vi "OX v1.2.vi"(2 "INDICATOR INPUT":dbl[](array[numeric]), 3 "DATA INPUT":dbl[](array[numeric])) -> (0 "OUTPUT":dbl[][](array[numeric]))   [LabVIEW 2019]
uses:
  <vilib>/ptbypt/NI_PtbyPt.lvlib
panel:
  in  "FU BUTTON FEEDBACK":dbl[](array[numeric])
  out "PH LED 6":bool=TRUE
  in  "PH CHECK 6":bool
  out "PH IND 6":bool=TRUE
  out "PH LED 5":bool=TRUE
  out "PH LED 4":bool=TRUE
  out "PH LED 3":bool=TRUE
  out "PH LED 2":bool=TRUE
  out "PH LED 1":bool=TRUE
  in  "PH CHECK 1":bool
  in  "PH CHECK 2":bool
  in  "PH CHECK 3":bool
  in  "PH CHECK 4":bool
  in  "PH CHECK 5":bool
  out "PH IND 5":bool=TRUE
  out "PH IND 4":bool=TRUE
  out "PH IND 3":bool=TRUE
  out "PH IND 2":bool=TRUE
  out "PH IND 1":bool=TRUE
  out "STARTUP GNG":bool=TRUE
  out "STARTUP GNG NUM":dbl
  out "STARTUP GNG LED":bool=TRUE
  out "CHILL GNG":bool=TRUE
  out "CHILL GNG NUM":dbl
  out "CHILL GNG LED":bool=TRUE
  out "OX ISO GNG":bool=TRUE
  out "OX ISO GNG NUM":dbl
  out "OX ISO GNG LED":bool=TRUE
  out "RECORD GNG":bool=TRUE
  out "RECORD GNG NUM":dbl
  out "RECORD GNG LED":bool=TRUE
  out "OX VENT GNG":bool=TRUE
  out "OX VENT GNG NUM":dbl
  out "OX VENT GNG LED":bool=TRUE
  out "OX CHILL LINE TEMP":dbl(slide) scale=-200.0..75.0
  out "OX CHILL RELIEF TEMP":dbl(slide) scale=-200.0..75.0
  out "OX TANK TEMP 4":dbl
  out "OX TANK TEMP 3":dbl
  out "OX TANK TEMP 2":dbl
  out "OX TANK TEMP 1":dbl
  out "OX MAIN VALVE TEMP":dbl(slide) scale=-200.0..75.0
  out "OX VENTURI TEMP":dbl(slide) scale=-200.0..75.0
  out "TANK TEMP CB 1":u32(colorbox)
  out "TANK TEMP CB 2":u32(colorbox)
  out "TANK TEMP CB 3":u32(colorbox)
  out "TANK TEMP CB 4":u32(colorbox)
  out "OX MAIN LINE TEMP":dbl(slide) scale=-200.0..75.0
  out "SUB PANELS GNG":bool=TRUE
  out "SUB PANEL OX GNG NUM":dbl
  out "SUB PANEL OX GNG LED":bool=TRUE
  out "VALVE STATES GNG":bool=TRUE
  out "VALVE ST OX GNG NUM":dbl
  out "VALVE ST OX GNG LED":bool=TRUE
  out "PRESS VALVES GNG":bool=TRUE
  out "PRESS VALVE OX GNG NUM":dbl
  out "PRESS VALVE OX GNG LED":bool=TRUE
  out "ARM GNG":bool=TRUE
  out "IGN TRIPPED GNG":bool=TRUE
  out "ARMED GNG NUM":dbl
  out "ARMED GNG LED":bool=TRUE
  out "IGN TRIPPED GNG NUM":dbl
  out "IGN TRIPPED GNG LED":bool=TRUE
  in  "Ox GNG BUTTON":bool
  out "OX GNG MAIN LED":bool=TRUE
  in  "ABORT BUTTON":bool
  out "ARMED PANEL LED":bool
  out "IGN INSERTED PANEL LED":bool
  out "NANNY PAN LED":bool
  out "SYS STATUS MAIN STRING":string
  out "REG PRESS GNG":bool=TRUE
  out "RELIEF GNG":bool=TRUE
  out "REG PRESS OX GNG NUM":dbl
  out "REG PRESS OX GNG LED":bool=TRUE
  out "RELIEF OX GNG NUM":dbl
  out "RELIEF OX GNG LED":bool=TRUE
  out "TANK PRESS GNG":bool=TRUE
  out "TANK PRESS OX GNG NUM":dbl
  out "TANK PRESS OX GNG LED":bool=TRUE
  out "FILL VALVES GNG":bool=TRUE
  out "FILL VALVE OX GNG NUM":dbl
  out "FILL VALVE OX GNG LED":bool=TRUE
  out "TANK LEVEL GNG":bool=TRUE
  out "TANK LEVEL OX GNG NUM":dbl
  out "TANK LEVEL OX GNG LED":bool=TRUE
  out "OX TANK RELIEF TEMP":dbl(slide) scale=-200.0..75.0
  out "MAIN PRESS OX METER":dbl(knob) scale=0.0..1600.0
  out "MAIN LINE PRESS OX METER":dbl(knob) scale=0.0..1600.0
  out "TANK PRESS OX METER":dbl(knob) scale=0.0..1600.0
  out "REG PRESS OX METER":dbl(knob) scale=0.0..1600.0
  out "Ox SYSTEM PRESSURE":dbl[](graph) caption="Waveform Chart - dark"
  out "FUEL TANK LEVEL (%)":dbl(slide) scale=0.0..100.0
  in  "ABV-OX-250  (Ox FILL)":bool
  out "OX FILL LED":bool=TRUE
  in  "ABV-OX-240 (Ox CHILL)":bool
  out "ABV-OX-240 LED":bool=TRUE
  in  "ABV-OX-230 (Ox MAIN)":bool
  out "ABV-OX-230 LED":bool=TRUE
  in  "ABV-OX-220 (Ox ISO)":bool
  out "ABV-OX-230 LED":bool=TRUE
  in  "ABV-OX-210 (Ox VENT)":bool
  out "ABV-OX-210 LED":bool=TRUE
  in  "ABV-OX-110 (Ox PRESS)":bool
  out "ABV-PR-110 LED":bool=TRUE
  # "Ox CONTROL"
  # "NANNY"
  # "IGNITOR \nINSERTED"
  # "ARMED"
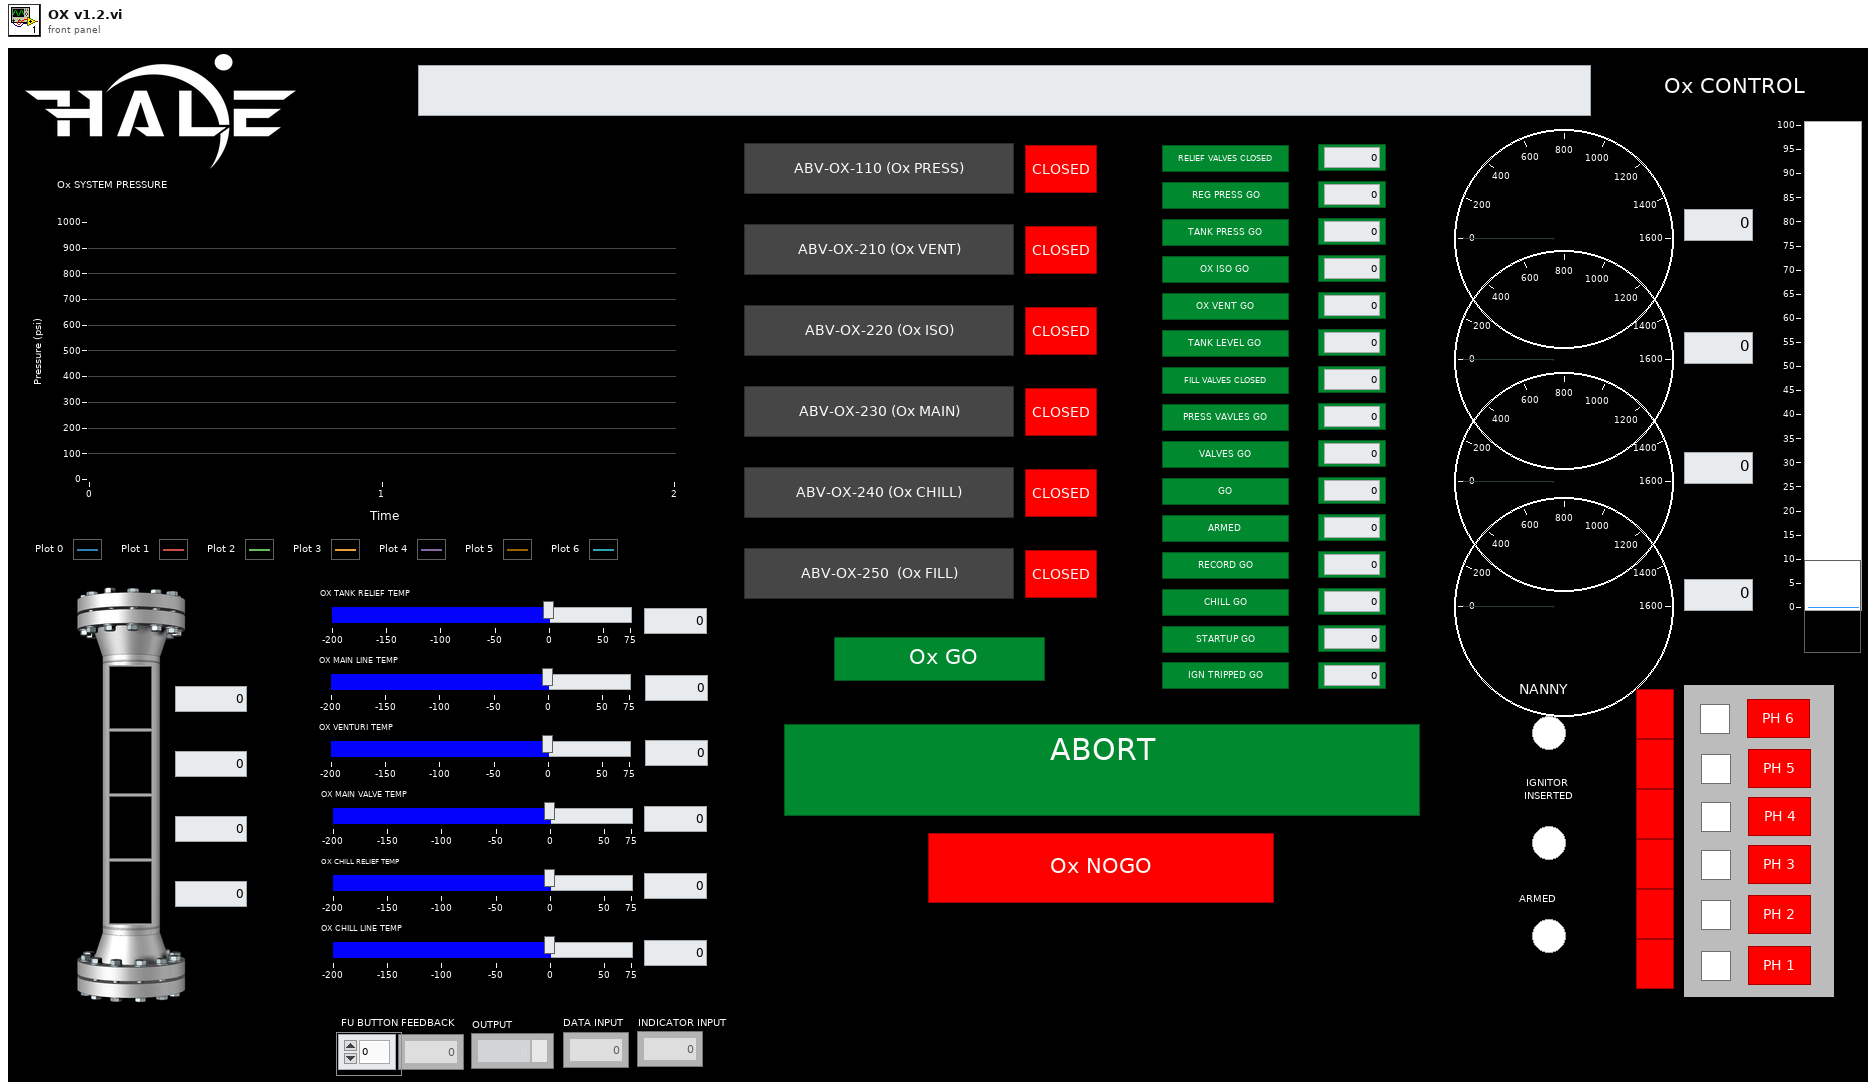
[diagram p1: front panel]
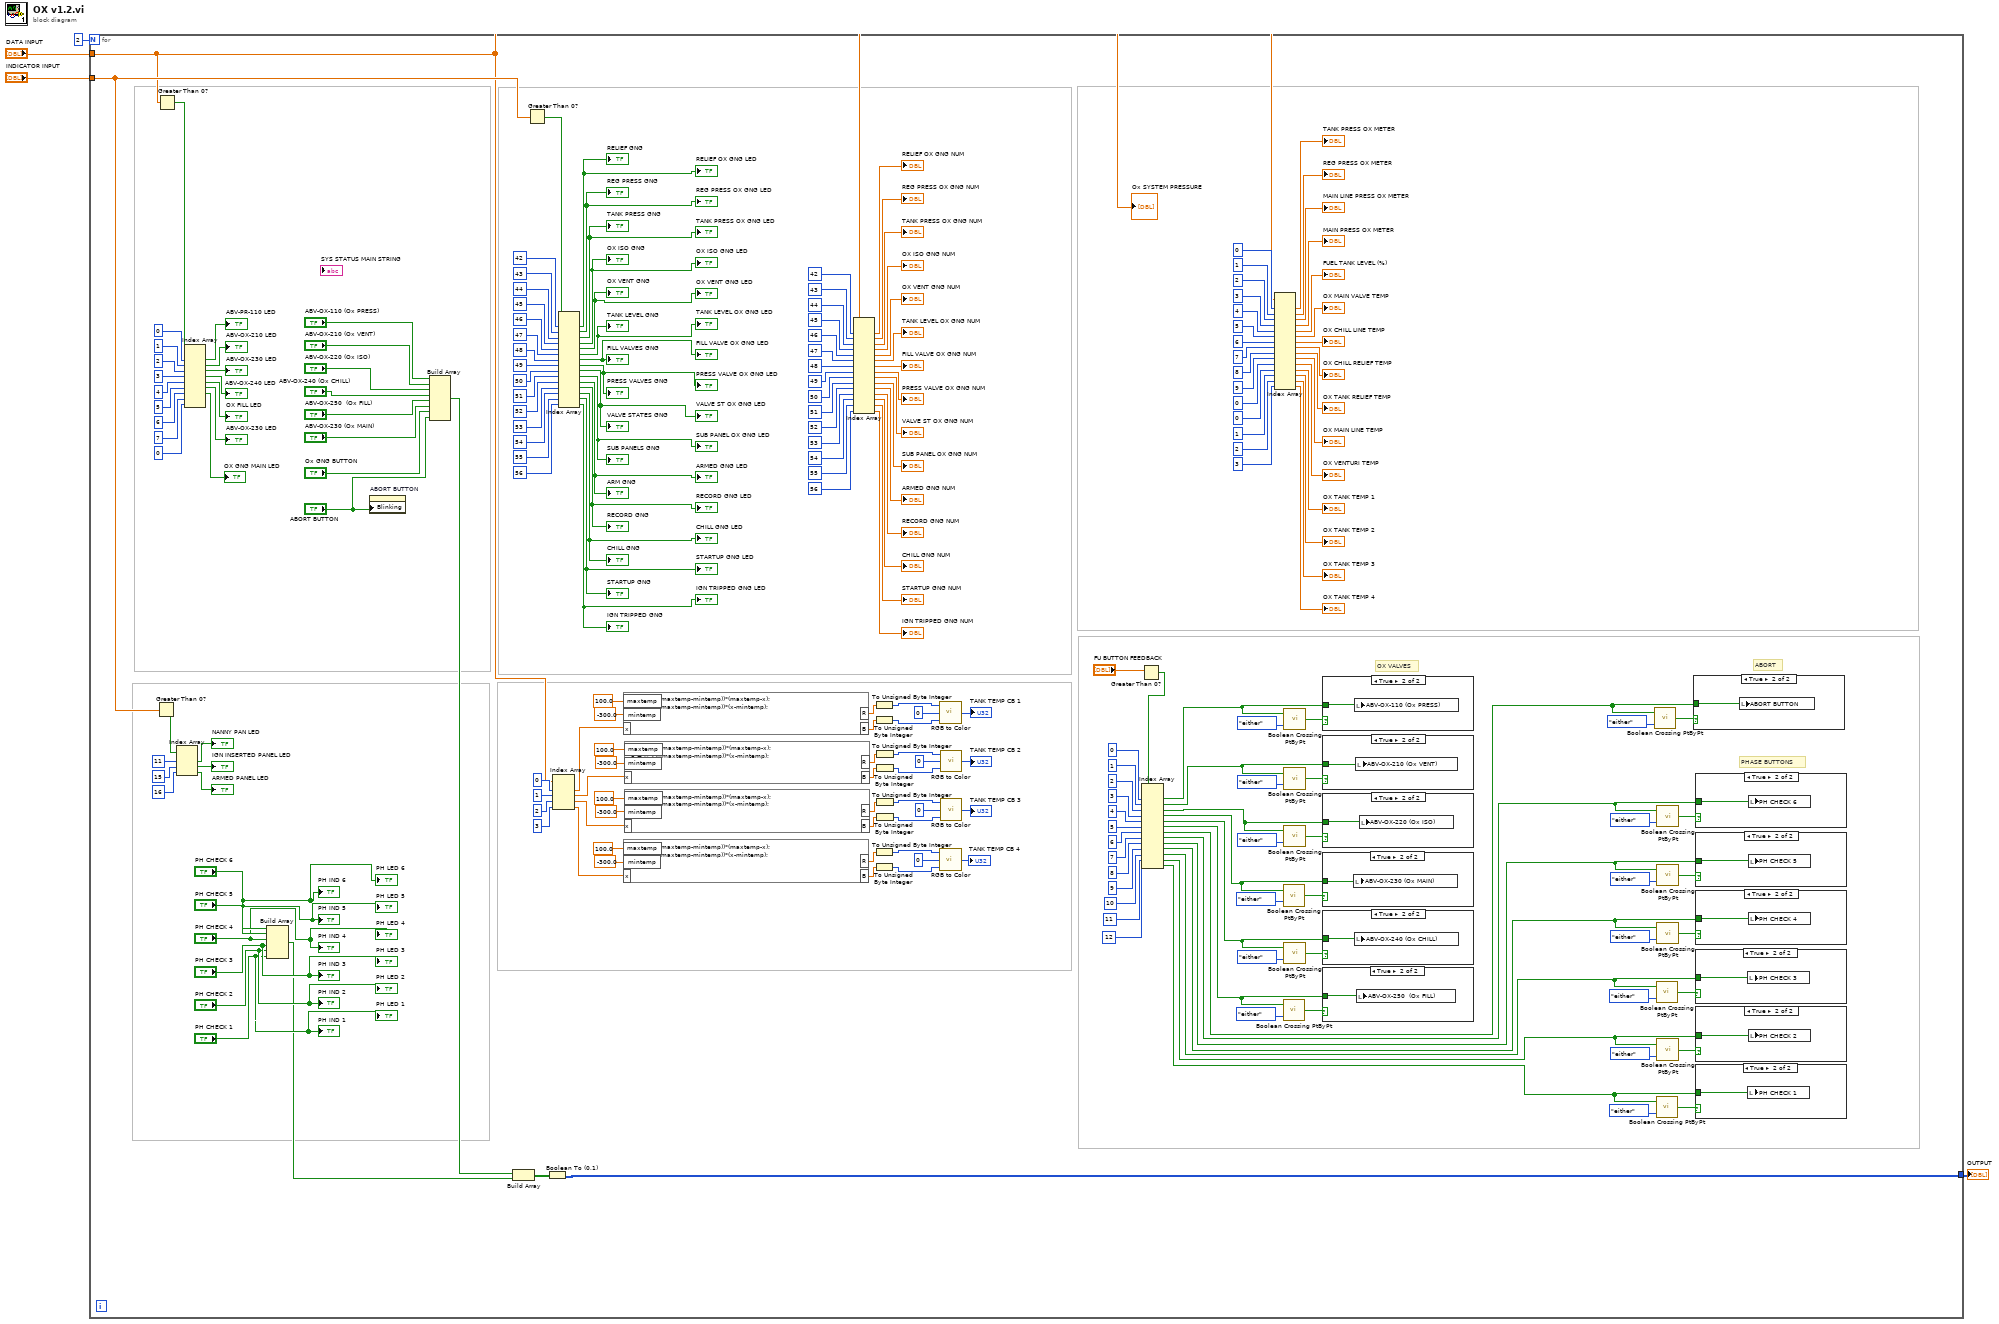
[diagram p0: block diagram]
diagram:
  n1 = for {
    N: 2 -> [_]
    tunnel: "INDICATOR INPUT" -> [w75]
    tunnel: "DATA INPUT" -> [w5]
    tunnel: [w64] -> w1
    # "ABORT"
    # "PHASE BUTTONS"
    # "OX VALVES"
    n2 = Greater Than 0?(x=w75) -> (x > 0?=w74:bool[])
    n3 = Greater Than 0?(x=w5) -> (x > 0?=w166:bool[])
    n4 = Index Array(array=w74, index #1=11 ("index"), index #2=15 ("index"), index #3=16 ("index")) -> (element #1=→"NANNY PAN LED":bool, element #2=→"IGN INSERTED PANEL LED":bool, element #3=→"ARMED PANEL LED":bool)
    n5 = Index Array(array=w166, index #1=0 ("index"), index #2=1 ("index"), index #3=2 ("index"), index #4=3 ("index"), index #5=4 ("index"), index #6=5 ("index"), index #7=6 ("index"), index #8=7 ("index"), index #9=0 ("index")) -> (element #1=→"ABV-PR-110 LED":bool, element #2=→"ABV-OX-210 LED":bool, element #3=→"ABV-OX-230 LED":bool, element #4=→"ABV-OX-240 LED":bool, element #5=→"OX FILL LED":bool, element #6=→"ABV-OX-230 LED":bool, element #7=→"OX GNG MAIN LED":bool)  [unwired: 2 out]
    n6 = Build Array("PH CHECK 6", "PH CHECK 5", "PH CHECK 4", "PH CHECK 3", "PH CHECK 2", "PH CHECK 1") -> (w66:bool[])
    n7 = property on="ABORT BUTTON" class="Bool (strict)"("Blinking"="ABORT BUTTON") -> ()  [unwired: 2 in, 2 out]
    n8 = Build Array("ABV-OX-110 (Ox PRESS)", "ABV-OX-210 (Ox VENT)", "ABV-OX-220 (Ox ISO)", "ABV-OX-240 (Ox CHILL)", "ABV-OX-250  (Ox FILL)", "ABV-OX-230 (Ox MAIN)", "Ox GNG BUTTON", "ABORT BUTTON") -> (w65:bool[])
    n9 = Build Array(w65, w66) -> (w67:bool[][])
    n10 = Greater Than 0?(x=w75) -> (x > 0?=w106:bool[])
    n11 = Boolean To (0,1)(Boolean=w67) -> (0, 1=w64:i16[][])
    n12 = Index Array(array=w5, index #1=0 ("index"), index #2=1 ("index"), index #3=2 ("index"), index #4=3 ("index")) -> (element #1=w114:dbl, element #2=w113:dbl, element #3=w112:dbl, element #4=w111:dbl)
    n13 = Index Array(array=w106, index #1=42 ("index"), index #2=43 ("index"), index #3=44 ("index"), index #4=45 ("index"), index #5=46 ("index"), index #6=47 ("index"), index #7=48 ("index"), index #8=49 ("index"), index #9=50 ("index"), index #10=51 ("index"), index #11=52 ("index"), index #12=53 ("index"), index #13=54 ("index"), index #14=55 ("index"), index #15=56 ("index")) -> (element #1=→"RELIEF OX GNG LED" →"RELIEF GNG":bool, element #2=→"REG PRESS OX GNG LED" →"REG PRESS GNG":bool, element #3=→"TANK PRESS OX GNG LED" →"TANK PRESS GNG":bool, element #4=→"OX ISO GNG LED" →"OX ISO GNG":bool, element #5=→"OX VENT GNG LED" →"OX VENT GNG":bool, element #6=→"TANK LEVEL OX GNG LED" →"TANK LEVEL GNG":bool, element #7=→"FILL VALVE OX GNG LED" →"FILL VALVES GNG":bool, element #8=→"PRESS VALVE OX GNG LED" →"PRESS VALVES GNG":bool, element #9=→"VALVE ST OX GNG LED" →"VALVE STATES GNG":bool, element #10=→"SUB PANEL OX GNG LED" →"SUB PANELS GNG":bool, element #11=→"ARMED GNG LED" →"ARM GNG":bool, element #12=→"RECORD GNG LED" →"RECORD GNG":bool, element #13=→"CHILL GNG LED" →"CHILL GNG":bool, element #14=→"STARTUP GNG LED" →"STARTUP GNG":bool, element #15=→"IGN TRIPPED GNG LED" →"IGN TRIPPED GNG":bool)
    n14 = formula code="B = (255/(maxtemp-mintemp))*(maxtemp-x);\nR = (255/(maxtemp-mintemp))*(x-mintemp);"("maxtemp"=100.0 ("input variable"), "mintemp"=-300.0 ("input variable"), "x"=w114) -> ("B"=w160:dbl, "R"=w162:dbl)
    n15 = formula code="B = (255/(maxtemp-mintemp))*(maxtemp-x);\nR = (255/(maxtemp-mintemp))*(x-mintemp);"("maxtemp"=100.0 ("input variable"), "mintemp"=-300.0 ("input variable"), "x"=w111) -> ("B"=w124:dbl, "R"=w126:dbl)
    n16 = formula code="B = (255/(maxtemp-mintemp))*(maxtemp-x);\nR = (255/(maxtemp-mintemp))*(x-mintemp);"("maxtemp"=100.0 ("input variable"), "mintemp"=-300.0 ("input variable"), "x"=w113) -> ("B"=w138:dbl, "R"=w140:dbl)
    n17 = formula code="B = (255/(maxtemp-mintemp))*(maxtemp-x);\nR = (255/(maxtemp-mintemp))*(x-mintemp);"("maxtemp"=100.0 ("input variable"), "mintemp"=-300.0 ("input variable"), "x"=w112) -> ("B"=w131:dbl, "R"=w133:dbl)
    n18 = Index Array(array=w5, index #1=42 ("index"), index #2=43 ("index"), index #3=44 ("index"), index #4=45 ("index"), index #5=46 ("index"), index #6=47 ("index"), index #7=48 ("index"), index #8=49 ("index"), index #9=50 ("index"), index #10=51 ("index"), index #11=52 ("index"), index #12=53 ("index"), index #13=54 ("index"), index #14=55 ("index"), index #15=56 ("index")) -> (element #1=→"RELIEF OX GNG NUM":dbl, element #2=→"REG PRESS OX GNG NUM":dbl, element #3=→"TANK PRESS OX GNG NUM":dbl, element #4=→"OX ISO GNG NUM":dbl, element #5=→"OX VENT GNG NUM":dbl, element #6=→"TANK LEVEL OX GNG NUM":dbl, element #7=→"FILL VALVE OX GNG NUM":dbl, element #8=→"PRESS VALVE OX GNG NUM":dbl, element #9=→"VALVE ST OX GNG NUM":dbl, element #10=→"SUB PANEL OX GNG NUM":dbl, element #11=→"ARMED GNG NUM":dbl, element #12=→"RECORD GNG NUM":dbl, element #13=→"CHILL GNG NUM":dbl, element #14=→"STARTUP GNG NUM":dbl, element #15=→"IGN TRIPPED GNG NUM":dbl)
    n19 = To Unsigned Byte Integer(number=w162) -> (unsigned 8bit integer=w161:u8)
    n20 = To Unsigned Byte Integer(number=w160) -> (unsigned 8bit integer=w159:u8)
    n21 = To Unsigned Byte Integer(number=w126) -> (unsigned 8bit integer=w125:u8)
    n22 = To Unsigned Byte Integer(number=w124) -> (unsigned 8bit integer=w123:u8)
    n23 = To Unsigned Byte Integer(number=w140) -> (unsigned 8bit integer=w139:u8)
    n24 = To Unsigned Byte Integer(number=w138) -> (unsigned 8bit integer=w137:u8)
    n25 = To Unsigned Byte Integer(number=w133) -> (unsigned 8bit integer=w132:u8)
    n26 = To Unsigned Byte Integer(number=w131) -> (unsigned 8bit integer=w130:u8)
    n27 = call <vilib>:"RGB to Color.vi"("B"=w159, "G"=u8 0, "R"=w161) -> ("Color"=→"TANK TEMP CB 1":u32)
    n28 = call <vilib>:"RGB to Color.vi"("B"=w123, "G"=u8 0, "R"=w125) -> ("Color"=→"TANK TEMP CB 4":u32)
    n29 = call <vilib>:"RGB to Color.vi"("B"=w137, "G"=u8 0, "R"=w139) -> ("Color"=→"TANK TEMP CB 2":u32)
    n30 = call <vilib>:"RGB to Color.vi"("B"=w130, "G"=u8 0, "R"=w132) -> ("Color"=→"TANK TEMP CB 3":u32)
    n31 = Greater Than 0?(x="FU BUTTON FEEDBACK") -> (x > 0?=w10:bool[])
    n32 = Index Array(array=w10, index #1=0 ("index"), index #2=1 ("index"), index #3=2 ("index"), index #4=3 ("index"), index #5=4 ("index"), index #6=5 ("index"), index #7=6 ("index"), index #8=7 ("index"), index #9=8 ("index"), index #10=9 ("index"), index #11=10 ("index"), index #12=11 ("index"), index #13=12 ("index")) -> (element #1=w25:bool, element #2=w24:bool, element #3=w23:bool, element #4=w22:bool, element #5=w21:bool, element #6=w20:bool, element #7=w19:bool, element #8=w18:bool, element #9=w17:bool, element #10=w16:bool, element #11=w15:bool, element #12=w14:bool, element #13=w13:bool)
    n33 = Index Array(array=w5, index #1=0 ("index"), index #2=1 ("index"), index #3=2 ("index"), index #4=3 ("index"), index #5=4 ("index"), index #6=5 ("index"), index #7=6 ("index"), index #8=7 ("index"), index #9=8 ("index"), index #10=9 ("index"), index #11=0 ("index"), index #12=0 ("index"), index #13=1 ("index"), index #14=2 ("index"), index #15=3 ("index")) -> (element #1=→"TANK PRESS OX METER":dbl, element #2=→"REG PRESS OX METER":dbl, element #3=→"MAIN LINE PRESS OX METER":dbl, element #4=→"MAIN PRESS OX METER":dbl, element #5=→"FUEL TANK LEVEL (%)":dbl, element #6=→"OX MAIN VALVE TEMP":dbl, element #7=→"OX CHILL LINE TEMP":dbl, element #8=→"OX CHILL RELIEF TEMP":dbl, element #9=→"OX TANK RELIEF TEMP":dbl, element #10=→"OX MAIN LINE TEMP":dbl, element #11=→"OX VENTURI TEMP":dbl, element #12=→"OX TANK TEMP 1":dbl, element #13=→"OX TANK TEMP 2":dbl, element #14=→"OX TANK TEMP 3":dbl, element #15=→"OX TANK TEMP 4":dbl)
    n34 = call <vilib>:"Boolean Crossing PtByPt.vi"("direction"=enum16{"either", "false-true", "true-false"}."either", "input"=w22) -> ("crossing"=w57:bool)  [unwired: 1 in]
    n35 = call <vilib>:"Boolean Crossing PtByPt.vi"("direction"=enum16{"either", "false-true", "true-false"}."either", "input"=w20) -> ("crossing"=w53:bool)  [unwired: 1 in]
    n36 = call <vilib>:"Boolean Crossing PtByPt.vi"("direction"=enum16{"either", "false-true", "true-false"}."either", "input"=w25) -> ("crossing"=w63:bool)  [unwired: 1 in]
    n37 = call <vilib>:"Boolean Crossing PtByPt.vi"("direction"=enum16{"either", "false-true", "true-false"}."either", "input"=w24) -> ("crossing"=w61:bool)  [unwired: 1 in]
    n38 = call <vilib>:"Boolean Crossing PtByPt.vi"("direction"=enum16{"either", "false-true", "true-false"}."either", "input"=w23) -> ("crossing"=w59:bool)  [unwired: 1 in]
    n39 = call <vilib>:"Boolean Crossing PtByPt.vi"("direction"=enum16{"either", "false-true", "true-false"}."either", "input"=w21) -> ("crossing"=w55:bool)  [unwired: 1 in]
    n40 = case shown="True" w57 {
      tunnel: w22 -> [_ w243]
      frame False {
      }
      frame True {
        n41 = local write "ABV-OX-230 (Ox MAIN)"(w243) -> ()
      }
    }
    n42 = case shown="True" w53 {
      tunnel: w20 -> [_ w241]
      frame False {
      }
      frame True {
        n43 = local write "ABV-OX-250  (Ox FILL)"(w241) -> ()
      }
    }
    n44 = case shown="True" w63 {
      tunnel: w25 -> [_ w246]
      frame False {
      }
      frame True {
        n45 = local write "ABV-OX-110 (Ox PRESS)"(w246) -> ()
      }
    }
    n46 = case shown="True" w61 {
      tunnel: w24 -> [_ w245]
      frame False {
      }
      frame True {
        n47 = local write "ABV-OX-210 (Ox VENT)"(w245) -> ()
      }
    }
    n48 = case shown="True" w59 {
      tunnel: w23 -> [_ w244]
      frame False {
      }
      frame True {
        n49 = local write "ABV-OX-220 (Ox ISO)"(w244) -> ()
      }
    }
    n50 = case shown="True" w55 {
      tunnel: w21 -> [_ w242]
      frame False {
      }
      frame True {
        n51 = local write "ABV-OX-240 (Ox CHILL)"(w242) -> ()
      }
    }
    n52 = call <vilib>:"Boolean Crossing PtByPt.vi"("direction"=enum16{"either", "false-true", "true-false"}."either", "input"=w19) -> ("crossing"=w39:bool)  [unwired: 1 in]
    n53 = call <vilib>:"Boolean Crossing PtByPt.vi"("direction"=enum16{"either", "false-true", "true-false"}."either", "input"=w15) -> ("crossing"=w45:bool)  [unwired: 1 in]
    n54 = call <vilib>:"Boolean Crossing PtByPt.vi"("direction"=enum16{"either", "false-true", "true-false"}."either", "input"=w13) -> ("crossing"=w41:bool)  [unwired: 1 in]
    n55 = call <vilib>:"Boolean Crossing PtByPt.vi"("direction"=enum16{"either", "false-true", "true-false"}."either", "input"=w18) -> ("crossing"=w51:bool)  [unwired: 1 in]
    n56 = call <vilib>:"Boolean Crossing PtByPt.vi"("direction"=enum16{"either", "false-true", "true-false"}."either", "input"=w17) -> ("crossing"=w49:bool)  [unwired: 1 in]
    n57 = call <vilib>:"Boolean Crossing PtByPt.vi"("direction"=enum16{"either", "false-true", "true-false"}."either", "input"=w16) -> ("crossing"=w47:bool)  [unwired: 1 in]
    n58 = call <vilib>:"Boolean Crossing PtByPt.vi"("direction"=enum16{"either", "false-true", "true-false"}."either", "input"=w14) -> ("crossing"=w43:bool)  [unwired: 1 in]
    n59 = case shown="True" w39 {
      tunnel: w19 -> [_ w234]
      frame False {
      }
      frame True {
        n60 = local write "ABORT BUTTON"(w234) -> ()
      }
    }
    n61 = case shown="True" w45 {
      tunnel: w15 -> [_ w237]
      frame False {
      }
      frame True {
        n62 = local write "PH CHECK 3"(w237) -> ()
      }
    }
    n63 = case shown="True" w41 {
      tunnel: w13 -> [_ w235]
      frame False {
      }
      frame True {
        n64 = local write "PH CHECK 1"(w235) -> ()
      }
    }
    n65 = case shown="True" w51 {
      tunnel: w18 -> [_ w240]
      frame False {
      }
      frame True {
        n66 = local write "PH CHECK 6"(w240) -> ()
      }
    }
    n67 = case shown="True" w49 {
      tunnel: w17 -> [_ w239]
      frame False {
      }
      frame True {
        n68 = local write "PH CHECK 5"(w239) -> ()
      }
    }
    n69 = case shown="True" w47 {
      tunnel: w16 -> [_ w238]
      frame False {
      }
      frame True {
        n70 = local write "PH CHECK 4"(w238) -> ()
      }
    }
    n71 = case shown="True" w43 {
      tunnel: w14 -> [_ w236]
      frame False {
      }
      frame True {
        n72 = local write "PH CHECK 2"(w236) -> ()
      }
    }
    "Ox SYSTEM PRESSURE" <- w5
    "PH IND 1" <- "PH CHECK 1"
    "PH IND 2" <- "PH CHECK 2"
    "PH IND 3" <- "PH CHECK 3"
    "PH IND 4" <- "PH CHECK 4"
    "PH IND 5" <- "PH CHECK 5"
    "PH LED 1" <- "PH CHECK 1"
    "PH LED 2" <- "PH CHECK 2"
    "PH LED 3" <- "PH CHECK 3"
    "PH LED 4" <- "PH CHECK 4"
    "PH LED 5" <- "PH CHECK 5"
    "PH IND 6" <- "PH CHECK 6"
    "PH LED 6" <- "PH CHECK 6"
  }
  "OUTPUT" <- w1
